vi "Write Measurements.vi"(8 "error in (no error)":errorcluster, 10 "BaseMeasurements":T1, 11 "PacificPowerSource in":refnum<class "PacificPowerSource.lvclass">) -> (0 "error out":errorcluster, 3 "PacificPowerSource out":refnum<class "PacificPowerSource.lvclass">)   [LabVIEW 2018, in "AcPwrPlugins.lvlib" / "PacificPowerSource.lvclass"]
uses:
  PacificPowerSource.lvclass
  TypeDefs/Measurements.ctl
  PacificPowerSource.lvclass/PacificPowerSource.ctl
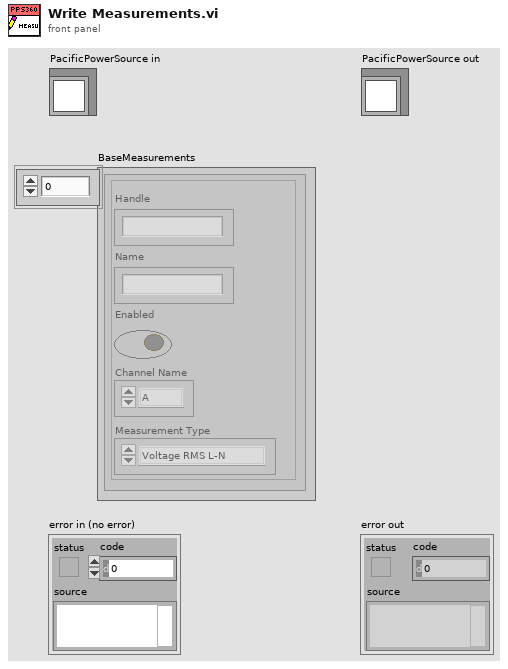
[diagram p1: front panel]
types:
  T1 = typedef "AcPwrPlugins.lvlib/PacificPowerSource.lvclass/Measurements.ctl" = cluster{"Handle":string, "Name":string, "Enabled ":bool, "Measurement Value":dbl, "Channel Name":enum16{"A", "B", "C"}, "Measurement Type ":enum16{"Voltage RMS L-N", "Voltage RMS L-L", "Frequency", "Current RMS", "Current Peak", "Crest Factor", "Power Factor", "Power VA", "Real Power"}}[]
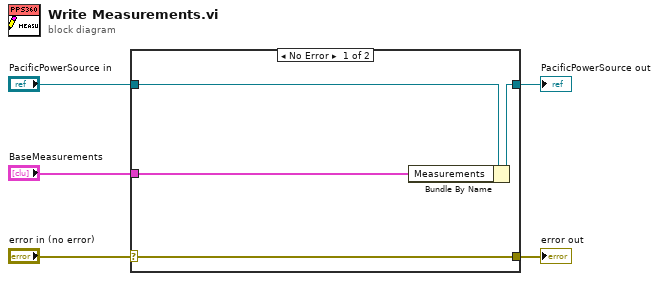
[diagram p0: block diagram]
diagram:
  n1 = case shown="No Error" "error in (no error)" {
    selector: "error in (no error)" -> [w9 w10]
    tunnel: [w9 w10] -> w4
    tunnel: [w7 w11] -> w2
    tunnel: "PacificPowerSource in" -> [w8 w11]
    tunnel: "BaseMeasurements" -> [w6 _]
    frame No Error {
      n2 = Bundle By Name(cluster=w8, "Measurements"=w6) -> (w7:refnum<class "PacificPowerSource.lvclass">)
    }
    frame Error {
    }
  }
  "error out" <- w4
  "PacificPowerSource out" <- w2
